vi "Swerve Motor Back Right.vi"(0 "Steer motor reference name":string="My Motor RefNum", 1 "Drive motor reference name":string="My Motor RefNum", 2 "Speed command":dbl, 3 "Direction command (deg)":dbl) -> ()   [LabVIEW 2018]
uses:
  <vilib>/Rock Robotics/WPI/ThirdParty/Phoenix-LabVIEW/Motor Controller/Controls/CTRE_Phoenix_MotorControl_ControlMode.ctl
  <vilib>/Rock Robotics/WPI/ThirdParty/Phoenix-LabVIEW/Motor Controller/Get/CTRE_Phoenix_MotorController_GetAnalogData.vi
  Robot Global Data.vi
  <vilib>/Rock Robotics/WPI/ThirdParty/REV Robotics/SPARK MAX/Typedef/Spark MAX Control Type.ctl
panel:
  in  "D-BL":dbl=0.5
  in  "I-BL":dbl=0.001
  in  "Ramp Rate-BL":dbl=60.0
  in  "I Zone-BL":dbl
  in  "F-BL":dbl=0.25
  in  "P-BL":dbl=4.0
  out "Veloicity":dbl
  out "Better Angle":dbl
  out "New Posiition":dbl
  out "Back Right Angle":dbl
  out "Position (Raw Sensor Units)":i32
  # "VI inputs"
  # "Intermediate values"
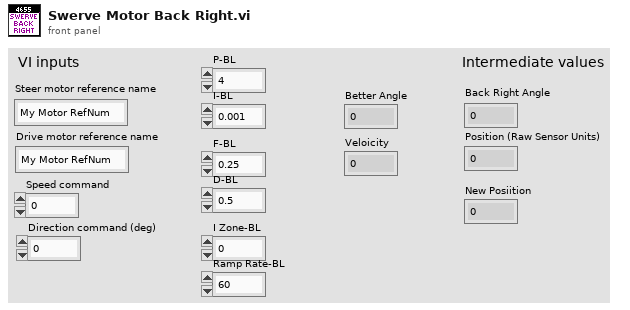
[diagram p1: front panel]
types:
  T1 = typedef "WPI_MotorControlDeviceRef.ctl" = cluster{"DeviceStatus":errorcluster, "Type":T2, "PWM":cluster{"PWM Channel":T3, "DeadBand":T4}, "CAN":cluster{"Device Number":u8, "SetOutput VI Ref":variant, "GetOutput VI Ref":variant, "Enable VI Ref":variant, "Disable VI Ref":variant, "Data":variant}, "Invert":bool, "DIO PWM":cluster{"PWM \"Enable\" Channel":T3, "DIOChannel":T5, "PWM Rate":dbl}}
  T2 = typedef "WPI_MotorControlType.ctl" = enum16{"PWM", "CAN", "DIO PWM"}
  T3 = typedef "FPGA_DIOPWMChannel.ctl" = enum8{"PWM 0", "PWM 1", "PWM 2", "PWM 3", "PWM 4", "PWM 5", "PWM 6", "PWM 7", "PWM 8", "PWM 9", "PWM MXP 0", "PWM MXP 1", "PWM MXP 2", "PWM MXP 3", "PWM MXP 4", "PWM MXP 5", "PWM MXP 6", "PWM MXP 7", "PWM MXP 8", "PWM MXP 9", "Invalid"}
  T4 = typedef "WPI_PWMDeadband.ctl" = cluster{"Name":string, "maxPositivePwm":i32, "minPositivePwm":i32, "centerPwm":i32, "maxNegativePwm":i32, "minNegativePwm":i32, "angularRange":u16}
  T5 = typedef "FPGA_DIOChannel.ctl" = enum8{"DIO 0", "DIO 1", "DIO 2", "DIO 3", "DIO 4", "DIO 5", "DIO 6", "DIO 7", "DIO 8", "DIO 9", "DIO MXP 0", "DIO MXP 1", "DIO MXP 2", "DIO MXP 3", "DIO MXP 4", "DIO MXP 5", "DIO MXP 6", "DIO MXP 7", "DIO MXP 8", "DIO MXP 9", "DIO MXP 10", "DIO MXP 11", "DIO MXP 12", "DIO MXP 13", "DIO MXP 14", "DIO MXP 15", "SPI Port CS1", "SPI Port CS2", "SPI Port CS3", "SPI Port MISO", "SPI Port MOSI", "Invalid"}
  T6 = typedef "Spark MAX Control Type.ctl" = enum16{"Percent VBus", "Voltage", "Velocity", "Position", "Smart Motion", "Current", "Smart Velocity"}
  T7 = typedef "CTRE_Phoenix_MotorControl_ControlMode.ctl" = u16
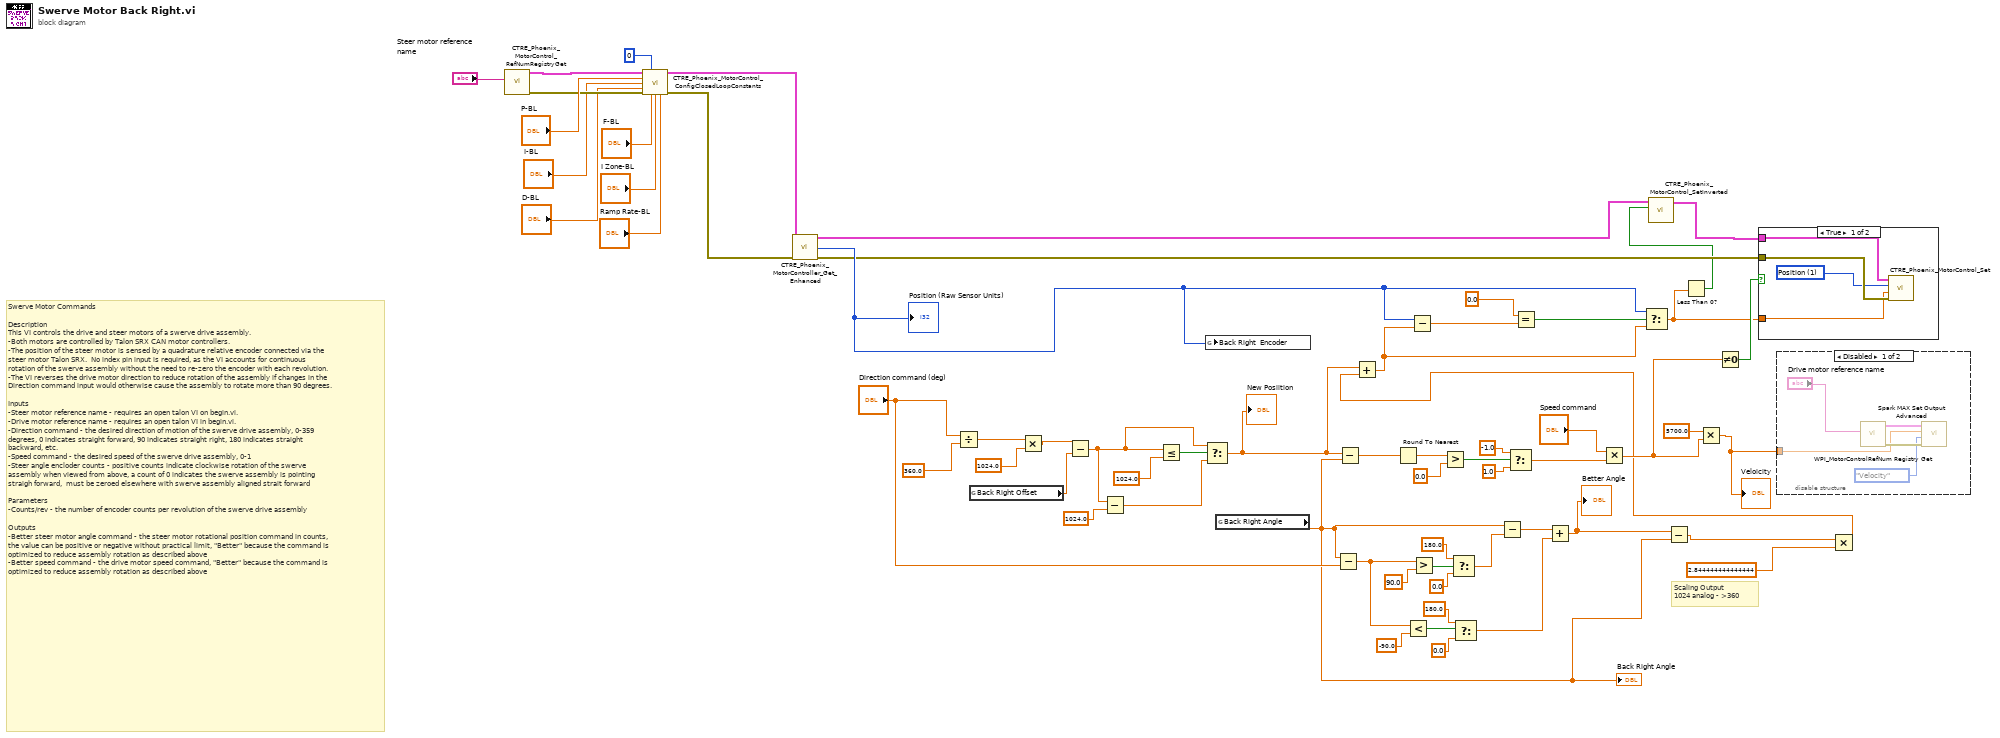
[diagram p0: block diagram]
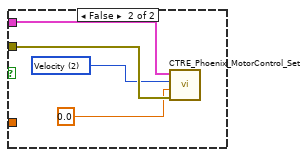
[diagram p3: hidden frame]
diagram:
  # "Scaling Output\n1024 analog - >360"
  # "Swerve Motor Commands\n\nDescription\nThis VI controls the drive and steer motors of a swerve drive assembly.  \n-Both motors are controlled by Talon SRX CAN motor controllers.  \n-The position of the steer motor is sensed by a quadrature relative encoder connected via the steer motor Talon SRX.  No index pin input is required, as the VI accounts for continuous rotation of the swerve assembly without the need to re-zero the encoder with each revolution.\n-The VI reverses the drive motor direction to reduce rotation of the assembly if changes in the Direction command input would otherwise cause the assembly to rotate more than 90 degrees.\n\nInputs\n-Steer motor reference name - requires an open talon VI on begin.vi.\n-Drive motor reference name - requires an open talon VI in begin.vi.\n-Direction command - the desired direction of motion of the swerve drive assembly, 0-359 degrees, 0 indicates straight forward, 90 indicates straight right, 180 indicates straight backward, etc.\n-Speed command - the desired speed of the swerve drive assembly, 0-1\n-Steer angle encloder counts - positive counts indicate clockwise rotation of the swerve assembly when viewed from above, a count of 0 indicates the swerve assembly is pointing straigh forward,  must be zeroed elsewhere with swerve assembly aligned strait forward\n\nParameters\n-Counts/rev - the number of encoder counts per revolution of the swerve drive assembly\n\nOutputs\n-Better steer motor angle command - the steer motor rotational position command in counts, the value can be positive or negative without practical limit, \"Better\" because the command is optimized to reduce assembly rotation as described above\n-Better speed command - the drive motor speed command, \"Better\" because the command is optimized to reduce assembly rotation as described above"
  n1 = call <vilib>:"CTRE_Phoenix_MotorControl_RefNumRegistryGet.vi"("refnum name"="Steer motor reference name") -> ("error out"=w7:errorcluster, "PhoenixMotorControlDevRef"=w10:T1)  [unwired: 9 in]
  n2 = call <vilib>:"CTRE_Phoenix_MotorControl_ConfigClosedLoopConstants.vi"("PhoenixMotorControlDevRef"=w10, "slotIdx"=0, "P"="P-BL", "I"="I-BL", "D"="D-BL", "error in (no error)"=w7, "F"="F-BL", "I Zone"="I Zone-BL", "timeoutMs"="Ramp Rate-BL") -> ("PhoenixMotorControlDevRef"=w9:T1, "error out"=w8:errorcluster)  [unwired: 5 in]
  n3 = call-poly <vilib>:"CTRE_Phoenix_MotorController_Get_Enhanced.vi"("PhoenixMotorControlDevRef"=w9, "error in"=w8) -> ("PhoenixMotorControlDevRef"=w4:T1, "AnalogInRaw"=w28:i32, "error out"=w24:errorcluster)  [unwired: 9 in, 2 out]
  "Position (Raw Sensor Units)" <- w28
  n4 = Divide(x="Direction command (deg)", y=360.0 ("x*y")) -> (x/y=w53:dbl)
  n5 = global read "Robot Global Data.vi" "Back Right Offset"() -> (w50:dbl)
  n6 = Multiply(x=w53, y=1024.0 ("x")) -> (x*y=w51:dbl)
  n7 = Subtract(x=w51, y=w50) -> (x-y=w45:dbl)
  n8 = Subtract(x=w45, y=1024.0 ("x")) -> (x-y=w46:dbl)
  n9 = Less Or Equal?(x=w45, y=1024.0 ("x")) -> (x <= y?=w47:bool)
  n10 = Select(t=w45, s=w47, f=w46) -> (s? t:f=w17:dbl)
  "New Posiition" <- w17
  n11 = global write "Robot Global Data.vi" "Back Right  Encoder"(w28) -> ()
  n12 = global read "Robot Global Data.vi" "Back Right Angle"() -> (w22:dbl)
  "Back Right Angle" <- w22
  n13 = Subtract(x=w22, y="Direction command (deg)") -> (x-y=w33:dbl)
  n14 = Subtract(x=w17, y=w22) -> (x-y=w57:dbl)
  n15 = Round To Nearest(number=w57) -> (nearest integer value=w59:dbl)
  n16 = Less?(x=w33, y=-90.0) -> (x < y?=w35:bool)
  n17 = Greater?(x=w33, y=90.0) -> (0:w42:bool)
  n18 = Greater?(x=w59, y=0.0) -> (0:w56:bool)
  n19 = Select(t=180.0, s=w42, f=0.0) -> (s? t:f=w38:dbl)
  n20 = Select(t=180.0, s=w35, f=0.0) -> (s? t:f=w31:dbl)
  n21 = Subtract(x=w22, y=w38) -> (x-y=w32:dbl)
  n22 = Select(t=-1.0, s=w56, f=1.0) -> (s? t:f=w44:dbl)
  n23 = Add(x=w32, y=w31) -> (x+y=w21:dbl)
  "Better Angle" <- w21
  n24 = Multiply(x="Speed command", y=w44) -> (x*y=w23:dbl)
  n25 = Subtract(x=w21, y=w22) -> (x-y=w19:dbl)
  n26 = Multiply(x=5700.0, y=w23) -> (x*y=w26:dbl)
  "Veloicity" <- w26
  n27 = Not Equal To 0?(x=w23) -> (x != 0?=w25:bool)
  n28 = disable-structure shown="Disabled" {
    disable-tunnel: w26 -> [w64 _]
    frame Disabled {
      n29 = call <vilib>:"WPI_MotorControlRefNum Registry Get.vi"("refnum name"="Drive motor reference name") -> ("error out"=w68:errorcluster, "MotorControlDevRef"=w67:T1)  [unwired: 9 in]
      n30 = call <vilib>:"Spark MAX Set Output Advanced.vi"("error in (no error)"=w68, "Control Mode"=Spark_MAX_Control_Type."Velocity", "Setpoint"=w64, "MotorControlDevRef"=w67) -> ()  [unwired: 6 in, 2 out]
    }
    frame Enabled {
    }
  }
  n31 = Multiply(x=w19, y=2.844444444444444) -> (x*y=w18:dbl)
  n32 = Add(x=w17, y=w18) -> (x+y=w16:dbl)
  n33 = Subtract(x=w28, y=w16) -> (x-y=w29:dbl)
  n34 = Equal?(x=0.0, y=w29) -> (x = y?=w55:bool)
  n35 = Select ("hold current steer angle\nif speed command is zero")(t=w28, s=w55, f=w16) -> (s? t:f=w2:dbl)
  n36 = Less Than 0?(x=w2) -> (x < 0?=w1:bool)
  n37 = call <vilib>:"CTRE_Phoenix_MotorControl_SetInverted.vi"("Invert?"=w1, "PhoenixMotorControlDevRef"=w4) -> ("PhoenixMotorControlDevRef"=w3:T1)  [unwired: 8 in, 1 out]
  n38 = case shown="True" w25 {
    tunnel: w3 -> [w72 w76]
    tunnel: w24 -> [w71 w75]
    tunnel: w2 -> [w70 _]
    frame True {
      w69 = T7 1 items=["PercentOutput"=0, "Position"=1, "Velocity"=2, "Current"=3, "Follower"=5, "MotionProfile"=6, "MotionMagic"=7, "MotionProfileArc"=10, "Disabled"=15] ("Control Mode")
      n39 = call <vilib>:"CTRE_Phoenix_MotorControl_Set.vi"("error in (no error)"=w71, "Output"=w70, "Control Mode"=w69, "PhoenixMotorControlDevRef"=w72) -> ()  [unwired: 6 in, 2 out]
    }
    frame False {
      w74 = T7 2 items=["PercentOutput"=0, "Position"=1, "Velocity"=2, "Current"=3, "Follower"=5, "MotionProfile"=6, "MotionMagic"=7, "MotionProfileArc"=10, "Disabled"=15] ("Control Mode")
      n40 = call <vilib>:"CTRE_Phoenix_MotorControl_Set.vi"("error in (no error)"=w75, "Output"=0.0 ("y"), "Control Mode"=w74, "PhoenixMotorControlDevRef"=w76) -> ()  [unwired: 6 in, 2 out]
    }
  }
